vi "CorrLast2ImgEdges.vi"() -> ()   [LabVIEW 2014]
uses:
  <vilib>/Analysis/2dsp.llb/2D Cross Correlation (DBL).vi
  <userlib>/Nanonis Prog Interface V5/Nanonis Prog Interface.lvlib
  <vilib>/Analysis/NI_AALPro.lvlib
panel:
  in  "method 2":u16(ring) items=["2nd Order Central", "4th Order Central", "Forward", "Backward"]
  out "Img1 3":picture
  in  "Direction (clockwise)":T1(ring)
  in  "method":T2(ring)
  out "Correl":picture
  out "pixel":i32=256
  out "Y drift":i32
  out "X drift":i32
  in  "First":i32=5 min=1 max=5
  in  "stop":bool
  in  "second":i32=4 min=0 max=5
  out "element 2":cluster{"last mod":timestamp, "path out":path}={"last mod"=timestamp(3554755212 s since 1904-01-01), "path out"=path "D:/STM Data/082016/160823_095600_2mol_chain/topo/160823_10-00-11_SPM001.sxm"}
  out "element":cluster{"last mod":timestamp, "path out":path}={"last mod"=timestamp(3554755074 s since 1904-01-01), "path out"=path "D:/STM Data/082016/160823_095600_2mol_chain/topo/160823_09-57-54_SPM001.sxm"}
  out "x-y":i32[](array[numeric])
  out "Img1 2":picture
  out "Img1":picture
  in  "Read channel 2":i8 min=-1
  in  "Path":path=path "D:/STM Data/082016/160823_095600_2mol_chain/topo"
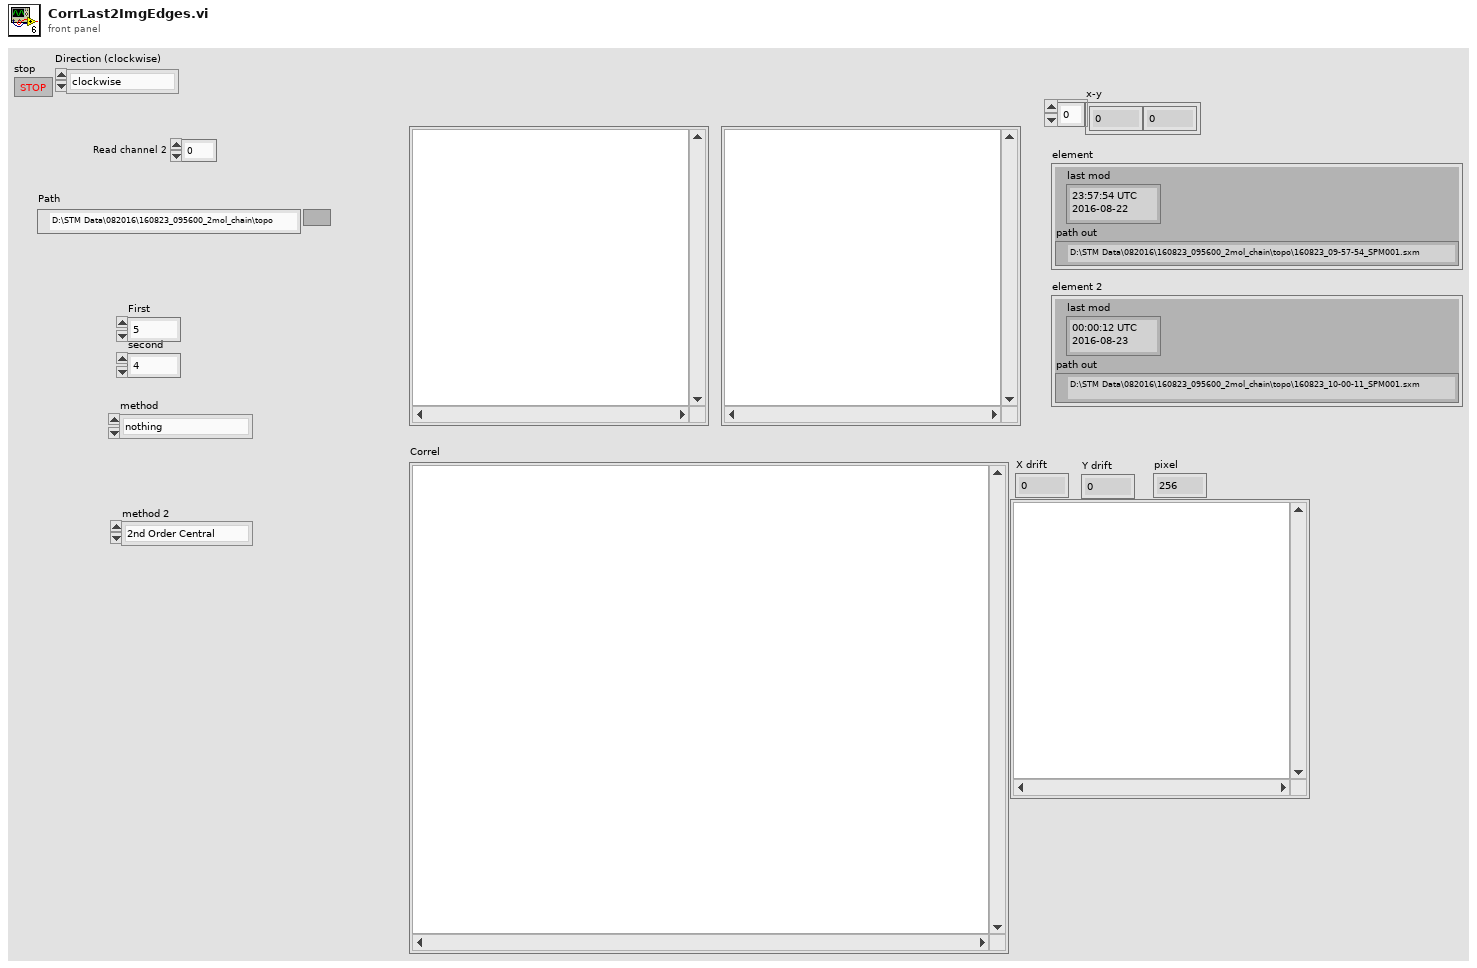
[diagram p1: front panel]
types:
  T1 = enum16{"clockwise", "counter-clockwise", "nothing"}
  T2 = enum16{"nothing", "average", "8bit", "average/plane", "minimum", "plane", "average/stddev", "plane/average"}
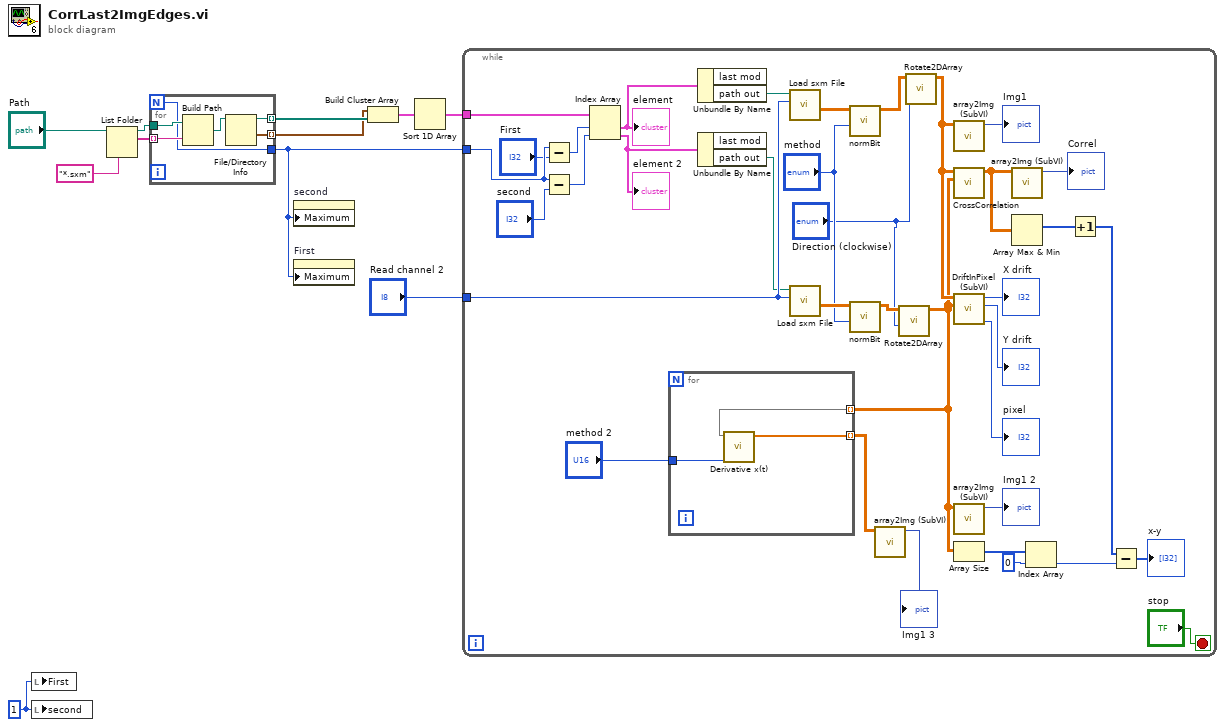
[diagram p0: block diagram]
diagram:
  w1 = 1 ("second")
  n1 = local write "First"(w1) -> ()
  n2 = local write "second"(w1) -> ()
  n3 = List Folder(path="Path", pattern="*.sxm") -> (path out=w8:path, filenames=w9:string[])  [unwired: 2 in, 2 out]
  n4 = for {
    N -> [w12]
    tunnel: w9 -> [w17] mode=indexing
    tunnel: w8 -> [w16]
    tunnel: [w14] -> w5 mode=indexing
    tunnel: [w13] -> w6 mode=indexing
    tunnel: [w12] -> w2
    n5 = Build Path(base path=w16, name or relative path=w17) -> (appended path=w15:path)
    n6 = File/Directory Info(path=w15) -> (path out=w13:path, last mod=w14:timestamp)  [unwired: 1 in, 5 out]
  }
  n7 = property on="second" class="DigNum (strict)"("Maximum"=w2) -> ()  [unwired: 2 in, 2 out]
  n8 = property on="First" class="DigNum (strict)"("Maximum"=w2) -> ()  [unwired: 2 in, 2 out]
  n9 = Build Cluster Array(w5, w6) -> (w4:cluster{"last mod":timestamp, "path out":path}[])
  n10 = Sort 1D Array(array=w4) -> (sorted array=w3:cluster{"last mod":timestamp, "path out":path}[])
  n11 = while {
    tunnel: "Read channel 2" -> [w53]
    tunnel: w3 -> [w44]
    tunnel: w2 -> [w37]
    stop <- "stop" stop-if-true
    n12 = Subtract(x=w37, y="First") -> (x-y=w39:i32)
    n13 = Subtract(x=w37, y="second") -> (x-y=w38:i32)
    n14 = Index Array(array=w44, index #1=w39, index #2=w38) -> (element #1=w43:cluster{"last mod":timestamp, "path out":path}, element #2=w41:cluster{"last mod":timestamp, "path out":path})
    "element" <- w43
    "element 2" <- w41
    n15 = Unbundle By Name(w43) -> ("path out"=w42:path)  [unwired: 1 out]
    n16 = Unbundle By Name(w41) -> ("path out"=w40:path)  [unwired: 1 out]
    n17 = call <userlib>:"Load sxm File.vi"("Read channel"=w53, "Scan data file"=w42) -> ("Data"=w33:sgl[][])  [unwired: 4 in, 5 out]
    n18 = call <userlib>:"Load sxm File.vi"("Read channel"=w53, "Scan data file"=w40) -> ("Data"=w32:sgl[][])  [unwired: 4 in, 5 out]
    n19 = call "normBit.vi"("method"="method", "Rxy"=w33) -> ("Array"=w25:dbl[][])  [unwired: 8 in, 1 out]
    n20 = call "normBit.vi"("method"="method", "Rxy"=w32) -> ("Array"=w23:dbl[][])  [unwired: 8 in, 1 out]
    n21 = call "Rotate2DArray.vi"("Direction (clockwise)"="Direction (clockwise)", "Array in"=w23) -> ("Array Out"=w21:dbl[][])  [unwired: 9 in]
    n22 = for {
      tunnel: w21 -> [w56] mode=indexing
      tunnel: [w55] -> w20 mode=indexing
      tunnel: "method 2" -> [w54]
      n23 = call <vilib>:"Derivative x(t).vi"("method"=w54, "X"=w56) -> ("dX/dt"=w55:dbl[])  [unwired: 8 in, 1 out]
    }
    n24 = call "array2Img (SubVI).vi"("Rxy"=w20) -> ("new picture"=→"Img1 3":picture)  [unwired: 10 in]
    n25 = call "Rotate2DArray.vi"("Direction (clockwise)"="Direction (clockwise)", "Array in"=w25) -> ("Array Out"=w24:dbl[][])  [unwired: 9 in]
    n26 = call "array2Img (SubVI).vi"("Rxy"=w24) -> ("new picture"=→"Img1":picture)  [unwired: 10 in]
    n27 = call-poly <vilib>:"CrossCorrelation.vi"("Y"=w21, "X"=w24) -> ("Rxy"=w28:dbl[][])  [unwired: 8 in, 1 out]
    n28 = call "DriftInPixel (SubVI).vi"("New image"=w21, "Ref image"=w24) -> ("pixel"=→"pixel":i32, "Y drift"=→"Y drift":i32, "X drift"=→"X drift":i32)  [unwired: 7 in]
    n29 = call "array2Img (SubVI).vi"("Rxy"=w21) -> ("new picture"=→"Img1 2":picture)  [unwired: 10 in]
    n30 = Array Size(array=w21) -> (size(s)=w49:i32[])
    n31 = call "array2Img (SubVI).vi"("Rxy"=w28) -> ("new picture"=→"Correl":picture)  [unwired: 10 in]
    n32 = Array Max & Min(array=w28) -> (max index (indices)=w50:i32[])  [unwired: 3 out]
    n33 = Index Array(array=w49, index=0) -> (element=w47:i32)
    n34 = Increment(x=w50) -> (x+1=w46:i32[])
    n35 = Subtract(x=w46, y=w47) -> (x-y=→"x-y":i32[])
  }
